vi "Example - Pop Up Blocking.vi"() -> ()   [LabVIEW 2016, in "SLL Debug.lvlib"]
uses:
  SLL Debug.lvlib
panel:
  in  "System Cluster":T1={"Numeric"=123.0, "Boolean"=TRUE, "String"="Hello World!", "System Array"=[0, 1, 2, 3]}
  # "Run this VI to see the SLL Blocking Pop Up VI in Action"
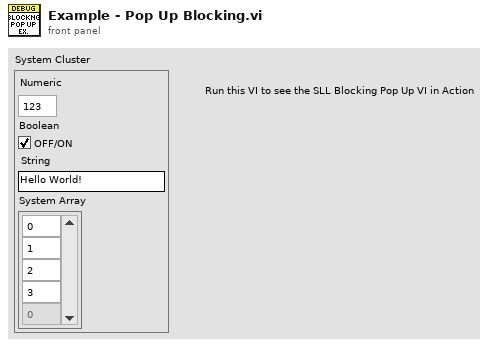
[diagram p1: front panel]
types:
  T1 = cluster{"Numeric":dbl, "Boolean":bool, "String":string, "System Array":u32[]}
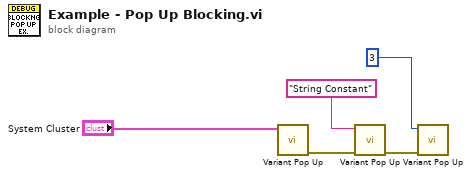
[diagram p0: block diagram]
diagram:
  n1 = call "Variant Pop Up.vi"("Variant"="System Cluster") -> ("error out"=w4:errorcluster)  [unwired: 10 in]
  n2 = call "Variant Pop Up.vi"("error in (no error)"=w4, "Variant"="String Constant") -> ("error out"=w2:errorcluster)  [unwired: 9 in]
  n3 = call "Variant Pop Up.vi"("error in (no error)"=w2, "Variant"=3) -> ()  [unwired: 9 in, 1 out]
